vi "1108_RobotDrivePantherDrive.vi"(6 "x-spin":dbl, 7 "Deadband":dbl, 8 "error in (no error)":errorcluster, 9 "y":dbl, 10 "x":dbl, 11 "RobotDriveDevRef":T1={"DevStatus"={"status"=FALSE, "code"=0, "source"=""}, "Motors[]"=[], "Square Inputs"=FALSE, "Max Output"=1.0}) -> (0 "error out":errorcluster, 2 "Motor Values":dbl[](array[numeric]), 3 "RobotDriveDevRef":T1={"DevStatus"={"status"=FALSE, "code"=0, "source"=""}, "Motors[]"=[], "Square Inputs"=FALSE, "Max Output"=1.0}, 4 "Motor angle":dbl)   [LabVIEW 2018]
doc: "Configures the motors for holonomic driving. Holonomic driving allows you to move the robot in any direction without first rotating or maneuvering the robot.\n\nThis VI requires the robot to have either four omni-directional wheels and four motors mounted at 45 degree angles in the four corners of a square frame or to have four mecanum wheels driven by four motors.\n\nThe control input is intended to come from autonomous code or any other time that polar notation is convenient.\n\nThis software is licensed. Open the labview\\readme\\WPI Robotics Library Open Source License.txt file for more information."
uses:
  <vilib>/Rock Robotics/WPI/RobotDrive/WPI_RobotDriveDevRef.ctl
  <vilib>/Rock Robotics/WPI/MotorControl/WPI_MotorControlDeviceRef.ctl
  <vilib>/Rock Robotics/WPI/MotorControl/WPI_MotorControlType.ctl
  <vilib>/Rock Robotics/SystemInterfaces/DIO/FPGA_DIOPWMChannel.ctl
  <vilib>/Rock Robotics/WPI/PWM/WPI_PWMDeadband.ctl
  <vilib>/Rock Robotics/SystemInterfaces/DIO/FPGA_DIOChannel.ctl
  <vilib>/Rock Robotics/SystemInterfaces/NetworkCommunication/NetComm_UsageReport_ResourceType.ctl
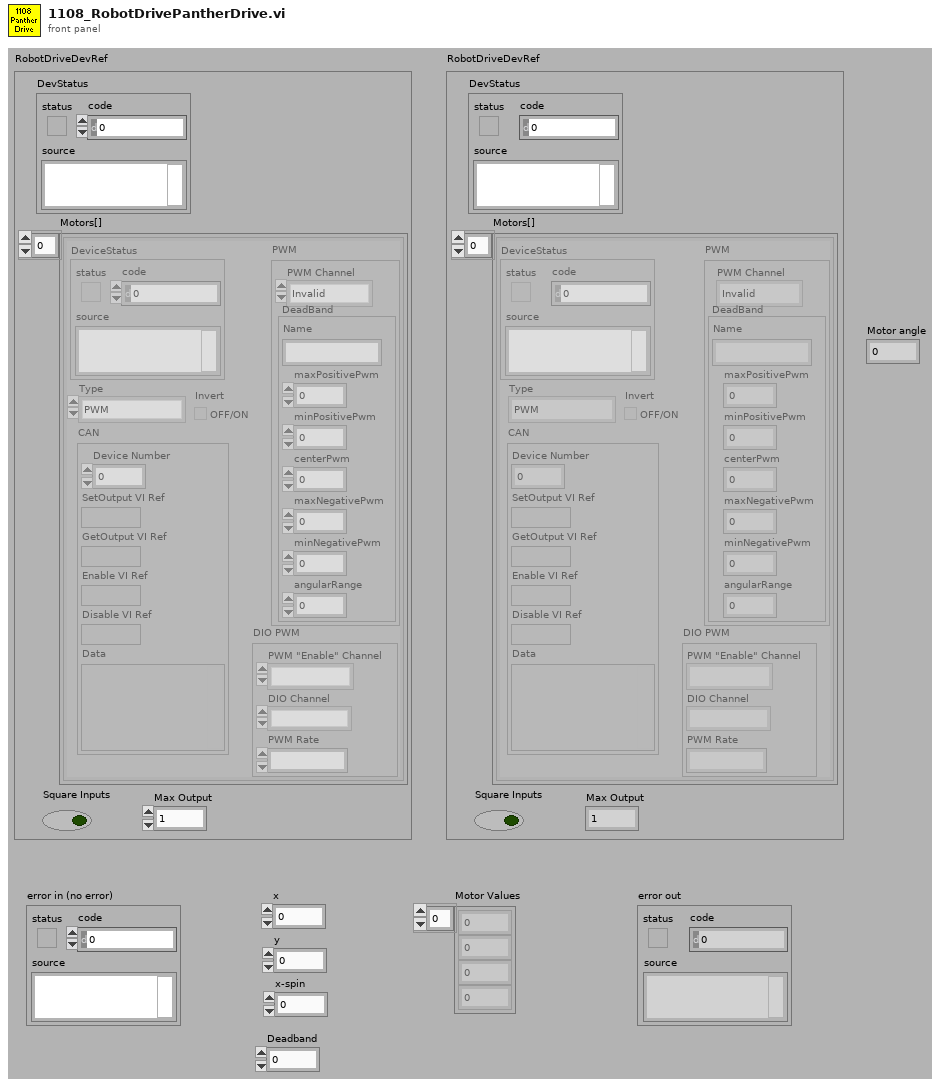
[diagram p1: front panel]
types:
  T1 = typedef "WPI_RobotDriveDevRef.ctl" = cluster{"DevStatus":errorcluster, "Motors[]":T2[], "Square Inputs":bool, "Max Output":dbl}
  T2 = typedef "WPI_MotorControlDeviceRef.ctl" = cluster{"DeviceStatus":errorcluster, "Type":T3, "PWM":cluster{"PWM Channel":T4, "DeadBand":T5}, "CAN":cluster{"Device Number":u8, "SetOutput VI Ref":variant, "GetOutput VI Ref":variant, "Enable VI Ref":variant, "Disable VI Ref":variant, "Data":variant}, "Invert":bool, "DIO PWM":cluster{"PWM \"Enable\" Channel":T4, "DIOChannel":T6, "PWM Rate":dbl}}
  T3 = typedef "WPI_MotorControlType.ctl" = enum16{"PWM", "CAN", "DIO PWM"}
  T4 = typedef "FPGA_DIOPWMChannel.ctl" = enum8{"PWM 0", "PWM 1", "PWM 2", "PWM 3", "PWM 4", "PWM 5", "PWM 6", "PWM 7", "PWM 8", "PWM 9", "PWM MXP 0", "PWM MXP 1", "PWM MXP 2", "PWM MXP 3", "PWM MXP 4", "PWM MXP 5", "PWM MXP 6", "PWM MXP 7", "PWM MXP 8", "PWM MXP 9", "Invalid"}
  T5 = typedef "WPI_PWMDeadband.ctl" = cluster{"Name":string, "maxPositivePwm":i32, "minPositivePwm":i32, "centerPwm":i32, "maxNegativePwm":i32, "minNegativePwm":i32, "angularRange":u16}
  T6 = typedef "FPGA_DIOChannel.ctl" = enum8{"DIO 0", "DIO 1", "DIO 2", "DIO 3", "DIO 4", "DIO 5", "DIO 6", "DIO 7", "DIO 8", "DIO 9", "DIO MXP 0", "DIO MXP 1", "DIO MXP 2", "DIO MXP 3", "DIO MXP 4", "DIO MXP 5", "DIO MXP 6", "DIO MXP 7", "DIO MXP 8", "DIO MXP 9", "DIO MXP 10", "DIO MXP 11", "DIO MXP 12", "DIO MXP 13", "DIO MXP 14", "DIO MXP 15", "SPI Port CS1", "SPI Port CS2", "SPI Port CS3", "SPI Port MISO", "SPI Port MOSI", "Invalid"}
  T7 = typedef "NetComm_UsageReport_ResourceType.ctl" = enum8{"Controller", "Module", "Language", "CANPlugin", "Accelerometer", "ADXL345", "AnalogChannel", "AnalogTrigger", "AnalogTriggerOutput", "CANJaguar", "Compressor", "Counter", "Dashboard", "DigitalInput", "DigitalOutput", "DriverStationCIO", "DriverStationEIO", "DriverStationLCD", "Encoder", "GearTooth", "Gyro", "I2C", "Framework", "Jaguar", "Joystick", "Kinect", "KinectStick", "PIDController", "Preferences", "PWM", "Relay", "RobotDrive", "SerialPort", "Servo", "Solenoid", "SPI", "Task", "Ultrasonic", "Victor", "Button", "Command", "AxisCamera", "PCVideoServer", "SmartDashboard", "Talon", "HiTechnicColorSensor", "HiTechnicAccel", "HiTechnicCompass", "SRF08", "AnalogOutput", "Victor SP", "Talon SRX", "CAN Talon SRX", "ADXL362 Accel", "ADXRS450 Gyro", "Rev SPARK", "Mindsensors SD540", "Digital Filter", "ADIS16448", "PDP", "PCM", "PigeonIMU", "Nidec Brushless", "CTRE CANifier", "CTRE Future 0", "CTRE Future 1", "CTRE Future 2", "CTRE Future 3", "CTRE Future 4", "CTRE Future 5", "CTRE Future 6", "Linear Filter", "Xbox Controller", "USB Camera", "NavX", "Pixy", "Pixy2", "ScanseSweep", "Shuffleboard", "CAN", "Digilent DMC60", "PWM Victor SPX", "Rev SPARK MAX PWM", "Rev SPARK MAX CAN", "ADIS16470"}
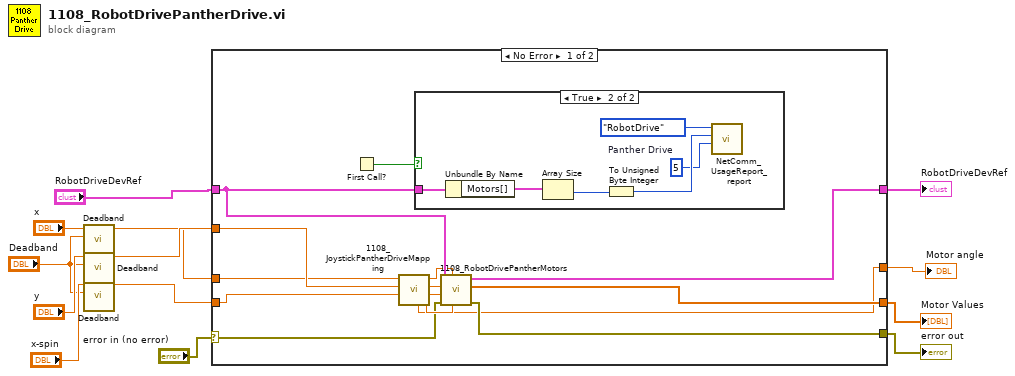
[diagram p0: block diagram]
diagram:
  n1 = call "Deadband.vi"("Deadband"="Deadband", "Input"="x") -> ("Output"=w4:dbl)  [unwired: 5 in]
  n2 = call "Deadband.vi"("Deadband"="Deadband", "Input"="y") -> ("Output"=w6:dbl)  [unwired: 5 in]
  n3 = call "Deadband.vi"("Deadband"="Deadband", "Input"="x-spin") -> ("Output"=w2:dbl)  [unwired: 5 in]
  n4 = case shown="No Error" "error in (no error)" {
    selector: "error in (no error)" -> [w22 w35]
    tunnel: w6 -> [w20 _]
    tunnel: w4 -> [w19 _]
    tunnel: "RobotDriveDevRef" -> [w21 w34]
    tunnel: [w24 w34] -> w11
    tunnel: [w25 w35] -> w10
    tunnel: w2 -> [w18 _]
    tunnel: [w26 _] -> w9
    tunnel: [w14 _] -> w8
    frame No Error {
      n5 = First Call?() -> (First Call?: T/F=w27:bool)
      n6 = call "1108_JoystickPantherDriveMapping.vi"("x-spin"=w18, "y"=w20, "x"=w19) -> ("Motor RR"=w23:dbl, "Motor FR"=w15:dbl, "Motor FL"=w16:dbl, "Motor RL"=w17:dbl, "theta"=w14:dbl)  [unwired: 4 in]
      n7 = case shown="True" w27 {
        tunnel: w21 -> [_ w28]
        frame False {
        }
        frame True {
          w31 = u8 5  # Panther Drive
          n8 = Unbundle By Name(w28) -> ("Motors[]"=w30:T2[])
          n9 = Array Size(array=w30) -> (size(s)=w29:i32)
          n10 = To Unsigned Byte Integer(number=w29) -> (unsigned 8bit integer=w32:u8)
          n11 = call <vilib>:"NetComm_UsageReport_report.vi"("Context"=w31, "Instance Number"=w32, "Resource Type"=NetComm_UsageReport_ResourceType."RobotDrive") -> ()  [unwired: 9 in]
        }
      }
      n12 = call "1108_RobotDrivePantherMotors.vi"("Rear Right"=w23, "Rear Left"=w17, "error in"=w22, "Front Right"=w15, "Front Left"=w16, "RobotDriveDevRef in"=w21) -> ("error out"=w25:errorcluster, "Motor Values"=w26:dbl[], "RobotDriveDevRef out"=w24:T1)  [unwired: 3 in]
    }
    frame Error {
    }
  }
  "error out" <- w10
  "RobotDriveDevRef" <- w11
  "Motor Values" <- w9
  "Motor angle" <- w8
